vi "Error Log.vi"(8 "error in (no error)":errorcluster) -> (0 "error out":errorcluster)   [LabVIEW 2017]
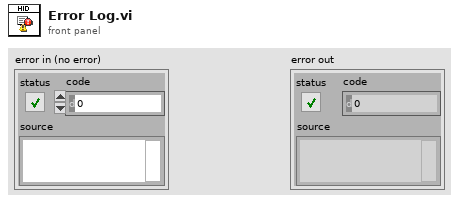
[diagram p1: front panel]
types:
  T1 = enum16{"open", "replace", "create", "open or create", "replace or create", "replace or create with confirmation"}
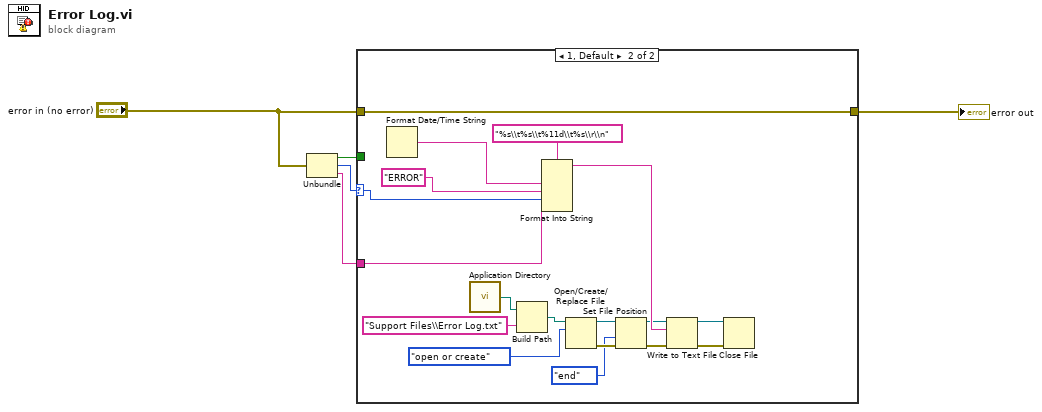
[diagram p0: block diagram]
diagram:
  n1 = Unbundle("error in (no error)") -> ("status"=w3:bool, "code"=w5:i32, "source"=w2:string)
  n2 = case shown="1, Default" w5 {
    selector: w5 -> [_ w9]
    tunnel: "error in (no error)" -> [w6 w23]
    tunnel: [w6 w23] -> w4
    tunnel: w3 -> [_ _]
    tunnel: w2 -> [_ w10]
    frame 0 {
    }
    frame 1, Default {
      n3 = Format Date/Time String() -> (date/time string=w7:string)  [unwired: 3 in]
      n4 = call <vilib>:"Application Directory.vi"() -> ("Application Directory"=w17:path)
      n5 = Build Path(base path=w17, name or relative path="Support Files\\Error Log.txt") -> (appended path=w18:path)
      n6 = Format Into String(format string="%s\\t%s\\t%11d\\t%s\\r\\n", w7, "ERROR", w9, w10) -> (resulting string=w19:string)  [unwired: 2 in, 1 out]
      n7 = Open/Create/Replace File(file path (use dialog)=w18, operation (0:open)=T1."open or create") -> (refnum out=w13:refnum<file>, error out=w20:errorcluster)  [unwired: 4 in, 1 out]
      n8 = Set File Position(refnum=w13, from (0:start)=enum16{"start", "end", "current"}."end", error in=w20) -> (refnum out=w12:refnum<file>, error out=w14:errorcluster)  [unwired: 1 in]
      n9 = Write to Text File(file (use dialog)=w12, text=w19, error in=w14) -> (refnum out=w21:refnum<file>, error out=w22:errorcluster)  [unwired: 1 in, 1 out]
      n10 = Close File(refnum=w21, error in=w22) -> ()  [unwired: 2 out]
    }
  }
  "error out" <- w4
